vi "EE_DataPreprocessingLoop.vi"(8 "StopButton Refnum":refnum<vi>, 10 "ChannelsDataNotifier in":T1, 11 "RawChannelsDataQueue in":T2) -> (2 "ChannelsDataNotifier out":T1, 3 "RawChannelsDataQueue out":T2)   [LabVIEW 2016, in "Emotiv Epoc.lvlib"]
uses:
  Emotiv Epoc.lvlib
  EE_Queue_Refnum.ctl
  EE_Queue_Data_Type.ctl
  EE_SignalStrength_enum.ctl
  EE_EEG_ContactQuality_enum.ctl
  EE_Notifier_Refnum.ctl
  EE_Notifier_Data_Type.ctl
  EE_DataChannels_enum.ctl
  EmotivEpocHeadsetControls.lvclass
panel:
  out "Renew Timestamp?":bool
  # "This VI is a part of BCI Design library, http://www.ru-bci.org \nCopyright © 2020, Sotnikov Peter, All rights reserved. License: CC BY-NC 4.0"
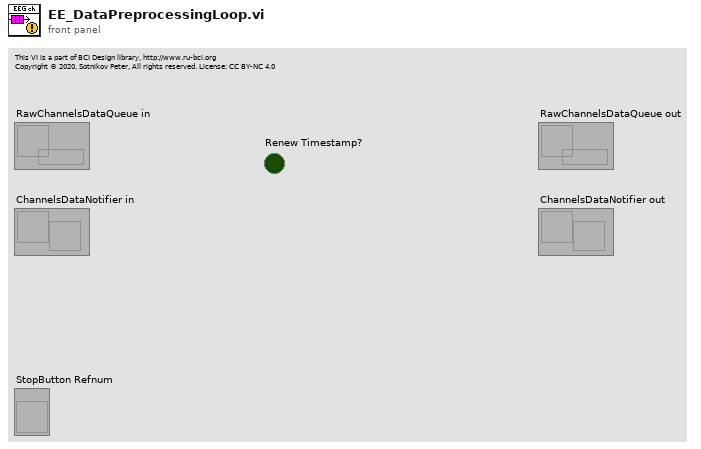
[diagram p1: front panel]
types:
  T1 = typedef "Emotiv Epoc.lvlib/EE_Notifier_Refnum.ctl" = refnum<notifier>
  T2 = typedef "Emotiv Epoc.lvlib/EE_Queue_Refnum.ctl" = refnum<queue>
  T3 = typedef "Emotiv Epoc.lvlib/EE_Notifier_Data_Type.ctl" = cluster{"EDK_Error":string, "Number of samples":u32, "Marker Waveform":waveform(dbl), "Array of EEG waveforms":waveform(dbl)[], "WirelessSignalStatus":T4, "EEG_ContactsQuality":T5[]}
  T4 = typedef "Emotiv Epoc.lvlib/EmotivEpocHeadsetControls.lvclass/EE_SignalStrength_enum.ctl" = enum32{"NO_SIGNAL", "BAD_SIGNAL", "GOOD_SIGNAL"}
  T5 = typedef "Emotiv Epoc.lvlib/EE_EEG_ContactQuality_enum.ctl" = enum16{"EEG_CQ_NO_SIGNAL", "EEG_CQ_VERY_BAD", "EEG_CQ_POOR", "EEG_CQ_FAIR", "EEG_CQ_GOOD"}
  T6 = typedef "Emotiv Epoc.lvlib/EmotivEpocHeadsetControls.lvclass/EE_DataChannels_enum.ctl" = enum32{"ED_COUNTER", "ED_INTERPOLATED", "ED_RAW_CQ", "ED_AF3", "ED_F7", "ED_F3", "ED_FC5", "ED_T7", "ED_P7", "ED_O1", "ED_O2", "ED_P8", "ED_T8", "ED_FC6", "ED_F4", "ED_F8", "ED_AF4", "ED_GYROX", "ED_GYROY", "ED_TIMESTAMP", "ED_ES_TIMESTAMP", "ED_FUNC_ID", "ED_FUNC_VALUE", "ED_MARKER", "ED_SYNC_SIGNAL"}
  T7 = typedef "Emotiv Epoc.lvlib/EE_Queue_Data_Type.ctl" = cluster{"FinishedLate?":bool, "UserActive?":bool, "WirelessSignalStatus":T4, "EDK_ERROR_CODE":i32, "nSampleOut":u32, "CurrentTimestamp":timestamp, "RawChannelsData ":dbl[][], "EEG_ContactsQuality":T5[]}
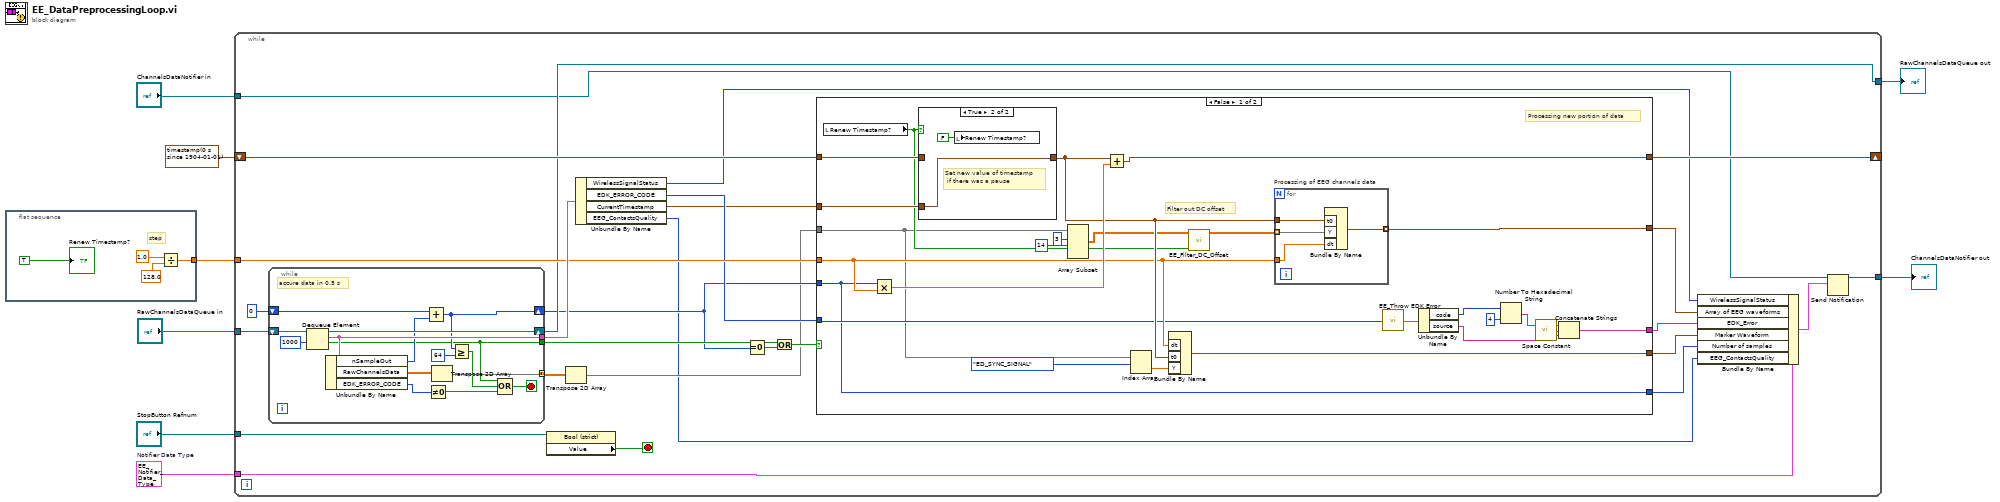
[diagram p0: block diagram]
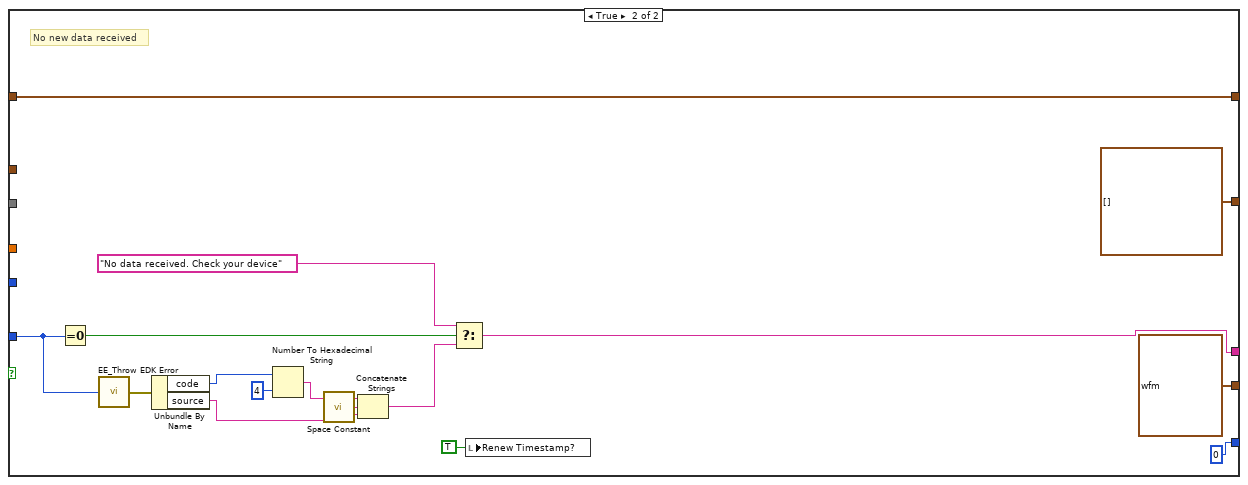
[diagram p3: hidden frame]
diagram:
  w2 = T3 {"EDK_Error"="", "Number of samples"=0, "Marker Waveform"={"t0"=timestamp(0 s since 1904-01-01), "dt"=1.0, "Y"=[]}, "Array of EEG waveforms"=[], "WirelessSignalStatus"=enum."NO_SIGNAL", "EEG_ContactsQuality"=[]}  # Notifier Data Type
  n1 = flat-sequence {
    tunnel: [w9] -> w7
    frame #0 {
      # "step"
      n2 = Divide(x=1.0, y=128.0) -> (x/y=w9:dbl)
      "Renew Timestamp?" <- TRUE ("Renew Timestamp?")
    }
  }
  n3 = while {
    tunnel: "RawChannelsDataQueue in" -> [w39]
    shift-right: [w35] -> _
    shift-left: timestamp(0 s since 1904-01-01) -> [w34]
    tunnel: w7 -> [w33]
    tunnel: "StopButton Refnum" -> [w31]
    tunnel: [w28] -> w4
    tunnel: "ChannelsDataNotifier in" -> [w27]
    tunnel: w2 -> [w26]
    tunnel: [w20] -> w1
    stop <- w30 stop-if-true
    n4 = while {
      tunnel: [w51] -> w38
      tunnel: [w42] -> w37
      shift-right: [w52] -> w28
      shift-left: w39 -> [w53]
      tunnel: [w49] -> w16 mode=concatenating
      shift-right: [w46] -> w17
      shift-left: u32 0 -> [w47]
      stop <- w44 stop-if-true
      # "accure data in 0.5 s"
      n5 = Dequeue Element(queue=w53, timeout in ms (-1)=1000) -> (queue out=w52:T2, element=w51:T7, timed out?=w42:bool)  [unwired: 1 in, 1 out]
      n6 = Unbundle By Name(w51) -> ("nSampleOut"=w48:u32, "RawChannelsData"=w50:dbl[][], "EDK_ERROR_CODE"=w41:i32)
      n7 = Add(x=w47, y=w48) -> (x+y=w46:u32)
      n8 = Not Equal To 0?(x=w41) -> (x != 0?=w40:bool)
      n9 = Transpose 2D Array(2D array=w50) -> (transposed array=w49:dbl[][])
      n10 = Greater Or Equal?(x=w46, y=u32 64) -> (x >= y?=w43:bool)
      n11 = Compound Arithmetic op=OR(w42, w43, w40) -> (w44:bool)
    }
    n12 = property class="Bool (strict)"(reference=w31) -> ("Value"=w30:bool)  [unwired: 1 in, 2 out]
    n13 = Transpose 2D Array(2D array=w16) -> (transposed array=w15:dbl[][])
    n14 = Unbundle By Name(w38) -> ("WirelessSignalStatus"=w23:T4, "EDK_ERROR_CODE"=w32:i32, "CurrentTimestamp"=w14:timestamp, "EEG_ContactsQuality"=w13:T5[])
    n15 = Equal To 0?(x=w17) -> (x = 0?=w29:bool)
    n16 = Or(x=w37, y=w29) -> (x .or. y?=w36:bool)
    n17 = case shown="False" w36 {
      tunnel: w15 -> [w58 _]
      tunnel: w14 -> [w78 _]
      tunnel: [w76 w101] -> w35
      tunnel: w34 -> [w79 w101]
      tunnel: w33 -> [w73 _]
      tunnel: w17 -> [w61 _]
      tunnel: [w72 waveform(dbl) {"t0"=timestamp(0 s since 1904-01-01), "dt"=1.0, "Y"=[]}] -> w24
      tunnel: [w71 waveform(dbl)[] []] -> w22
      tunnel: w32 -> [w64 w92]
      tunnel: [w63 w88] -> w25
      tunnel: [w61 u32 0 ("nSampleOut")] -> w19
      frame False {
        # "Filter out DC offset"
        # "Processing new portion of data"
        n18 = local read "Renew Timestamp?"() -> (w59:bool)
        n19 = Multiply(x=w61, y=w73) -> (x*y=w77:dbl)
        n20 = case shown="True" w59 {
          tunnel: w79 -> [w84 _]
          tunnel: [w84 w86] -> w75
          tunnel: w78 -> [_ w86]
          frame False {
          }
          frame True {
            # "Set new value of timestamp\n if there was a pause"
            n21 = local write "Renew Timestamp?"(FALSE ("Renew Timestamp?")) -> ()
          }
        }
        n22 = Array Subset(array=w58, index (row)=3 ("index"), length (row)=14 ("length")) -> (w57:dbl[][])  [unwired: 2 in]
        n23 = Add(x=w75, y=w77) -> (x+y=w76:timestamp)
        n24 = Index Array(array=w58, index (row)=EE_DataChannels_enum."ED_SYNC_SIGNAL" ("EE_DataChannels_enum")) -> (element=w74:dbl[])  [unwired: 1 in]
        n25 = Bundle By Name("dt"=w73, "t0"=w75, "Y"=w74) -> (w72:waveform(dbl))  [unwired: 1 in]
        n26 = call "EE_Filter_DC_Offset.vi"("Initialiaze?"=w59, "Raw Data In"=w57) -> ("Filtered Data out"=w60:dbl[][])  [unwired: 5 in]
        n27 = for "Processing of EEG channels data" {
          tunnel: w60 -> [w80] mode=indexing
          tunnel: w75 -> [w83]
          tunnel: w73 -> [w82]
          tunnel: [w81] -> w71 mode=indexing
          n28 = Bundle By Name("t0"=w83, "Y"=w80, "dt"=w82) -> (w81:waveform(dbl))  [unwired: 1 in]
        }
        n29 = call "EE_Throw EDK Error.vi"("edkErrorCode"=w64) -> ("edkErroCode"=w65:errorcluster)
        n30 = Unbundle By Name(w65) -> ("code"=w66:i32, "source"=w70:string)
        n31 = Number To Hexadecimal String(1:i16 4 ("width (-)"), 2:w66) -> (0:w68:string)
        n32 = call <vilib>:"Space Constant.vi"() -> ("String"=w69:string)
        n33 = Concatenate Strings(w68, w69, w70) -> (w63:string)
      }
      frame True {
        # "No new data received"
        n34 = Equal To 0?(x=w92) -> (x = 0?=w91:bool)
        n35 = call "EE_Throw EDK Error.vi"("edkErrorCode"=w92) -> ("edkErroCode"=w93:errorcluster)
        n36 = Unbundle By Name(w93) -> ("code"=w94:i32, "source"=w98:string)
        n37 = Number To Hexadecimal String(1:i16 4 ("width (-)"), 2:w94) -> (0:w96:string)
        n38 = call <vilib>:"Space Constant.vi"() -> ("String"=w97:string)
        n39 = Concatenate Strings(w96, w97, w98) -> (w89:string)
        n40 = Select(t="No data received. Check your device", s=w91, f=w89) -> (s? t:f=w88:string)
        n41 = local write "Renew Timestamp?"(TRUE ("Renew Timestamp?")) -> ()
      }
    }
    n42 = Bundle By Name(cluster=w26, "WirelessSignalStatus"=w23, "Array of EEG waveforms"=w22, "EDK_Error"=w25, "Marker Waveform"=w24, "Number of samples"=w19, "EEG_ContactsQuality"=w13) -> (w21:T3)
    n43 = Send Notification(notification=w21, notifier=w27) -> (notifier out=w20:T1)  [unwired: 1 in, 1 out]
  }
  "RawChannelsDataQueue out" <- w4
  "ChannelsDataNotifier out" <- w1
